vi "StateSpaceController.vi"(8 "u_Range":cluster{"u_max":dbl, "u_min":dbl}, 9 "goal_next":T1=[[-inf], [-inf]], 10 "x":T1=[[0.0], [0.0]], 11 "Gains":T2) -> (3 "u":dbl)   [LabVIEW 2017]
uses:
  <vilib>/Analysis/Matrix/Datatypes/RealMatrix.ctl
  <vilib>/Analysis/baseanly.llb/Real A x B.vi
  <vilib>/Analysis/Matrix/Numeric/Conversions/Matrix To Array - RM.vi
  <vilib>/Analysis/Matrix/Numeric/Conversions/Array To Matrix - RA2.vi
  <vilib>/Analysis/Matrix/Comparison/Equal/Equal - RM,RM.vi
  <vilib>/Analysis/Matrix/Numeric/Subtract/Subtract - RM,RM.vi
  <vilib>/Analysis/Matrix/Numeric/Multiply/Multiply - RM,RM.vi
  <vilib>/Analysis/Matrix/NI_Matrix.lvlib
  <vilib>/Analysis/NI_AALBase.lvlib
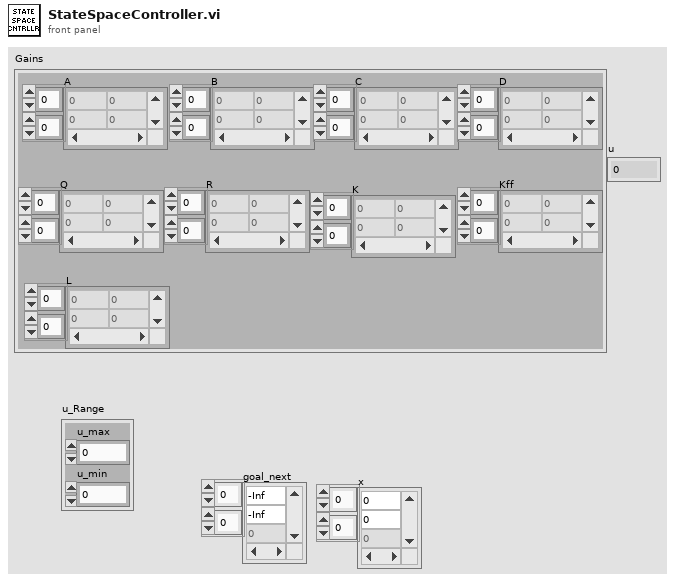
[diagram p1: front panel]
types:
  T1 = typedef "NI_Matrix.lvlib/RealMatrix.ctl" = dbl[][]
  T2 = cluster{"A":T1, "B":T1, "C":T1, "D":T1, "Q":T1, "R":T1, "K":T1, "Kff":T1, "L":T1}
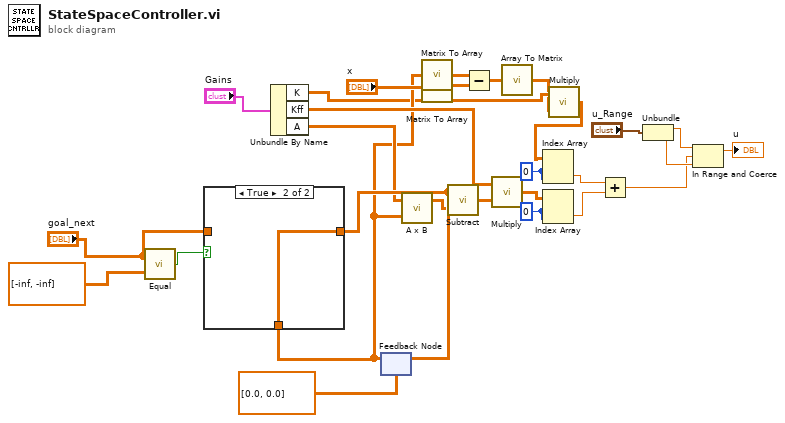
[diagram p0: block diagram]
diagram:
  w6 = 0 ("index (row)")
  w16 = 0 ("index (row)")
  n1 = call-poly <vilib>:"Equal.vi"("Real Matrix B"=T1 [[-inf], [-inf]], "Real Matrix A"="goal_next") -> ("A = B?"=w28:bool)
  n2 = Unbundle By Name("Gains") -> ("K"=w3:T1, "Kff"=w18:T1, "A"=w13:T1)
  n3 = feedback #1(T1 [[0.0], [0.0]] ("Real Matrix B")) -> (w7:T1)
  n4 = case shown="True" w28 {
    tunnel: [w29 w30] -> w14
    tunnel: "goal_next" -> [w29 _]
    tunnel: w7 -> [_ w30]
    frame False {
    }
    frame True {
    }
  }
  n5 = feedback-in #1(w14) -> ()
  n6 = call-poly <vilib>:"A x B.vi"("B"=w7, "A"=w13) -> ("A x B"=w12:T1)  [unwired: 1 out]
  n7 = call-poly <vilib>:"Matrix To Array.vi"("Real Matrix"=w7) -> ("Real 2D Array"=w11:dbl[][])
  n8 = call-poly <vilib>:"Matrix To Array.vi"("Real Matrix"="x") -> ("Real 2D Array"=w10:dbl[][])
  n9 = call-poly <vilib>:"Subtract.vi"("Real Matrix B"=w12, "Real Matrix A"=w14) -> ("A - B"=w19:T1)
  n10 = Subtract(x=w11, y=w10) -> (x-y=w9:dbl[][])
  n11 = call-poly <vilib>:"Multiply.vi"("Real Matrix B"=w19, "Real Matrix A"=w18) -> ("A * B"=w17:T1)
  n12 = call-poly <vilib>:"Array To Matrix.vi"("Real 2D Array"=w9) -> ("Real Matrix"=w2:T1)
  n13 = Index Array(array=w17, index (row)=w16, index (col)=w16) -> (element=w5:dbl)
  n14 = call-poly <vilib>:"Multiply.vi"("Real Matrix B"=w2, "Real Matrix A"=w3) -> ("A * B"=w1:T1)
  n15 = Index Array(array=w1, index (row)=w6, index (col)=w6) -> (element=w4:dbl)
  n16 = Add ("Add.vi")(x=w4, y=w5) -> (x+y=w15:dbl)
  n17 = Unbundle("u_Range") -> ("u_max"=w26:dbl, "u_min"=w25:dbl)
  n18 = In Range and Coerce(upper limit=w26, x=w15, lower limit=w25) -> (coerced(x)=→"u":dbl)  [unwired: 1 out]
